vi "Letter to Number.vi"(1 "Letter":string) -> (0 "Number":i32)   [LabVIEW 2019, in "Control Experiment.lvclass"]
uses:
  Control Experiment.lvclass
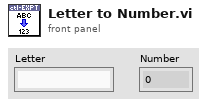
[diagram p1: front panel]
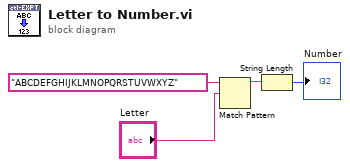
[diagram p0: block diagram]
diagram:
  n1 = Match Pattern(string="ABCDEFGHIJKLMNOPQRSTUVWXYZ", regular expression="Letter") -> (before substring=w2:string)  [unwired: 1 in, 3 out]
  n2 = String Length(string=w2) -> (length=→"Number":i32)
